vi "Add_Shortcut.vi"(8 "error in (no error)":errorcluster, 9 "shortcutAddresses":T1[](array[typedef]), 10 "shortcut":refnum<class "IB_Shortcut.lvclass">, 11 "IB_Source in":refnum<class "IB_Source.lvclass">) -> (0 "error out":errorcluster, 1 "name change?":bool, 2 "shortcut":refnum<class "IB_Shortcut.lvclass">, 3 "IB_Source out":refnum<class "IB_Source.lvclass">)   [LabVIEW 2020, in "IB_Source.lvclass"]
uses:
  <vilib>/AppBuilder/IB_Classes/Source/IB_Source.lvclass
  <vilib>/AppBuilder/IB_Classes/Source/IB_Source.lvclass/IB_Source.ctl
  <vilib>/AppBuilder/IB_Classes/Shortcut/IB_Shortcut.lvclass
  <resource>/Framework/Providers/Builds/Installer/CDK_sTypeDef_ShortcutAddress.ctl
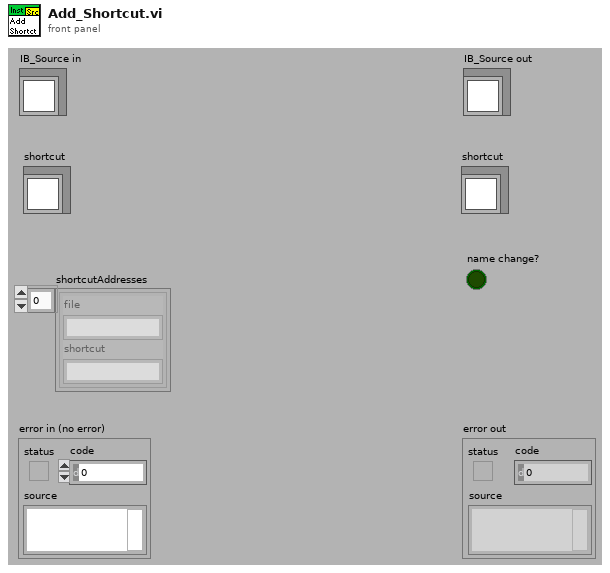
[diagram p1: front panel]
types:
  T1 = typedef "CDK_sTypeDef_ShortcutAddress.ctl" = cluster{"file":string, "shortcut":string}
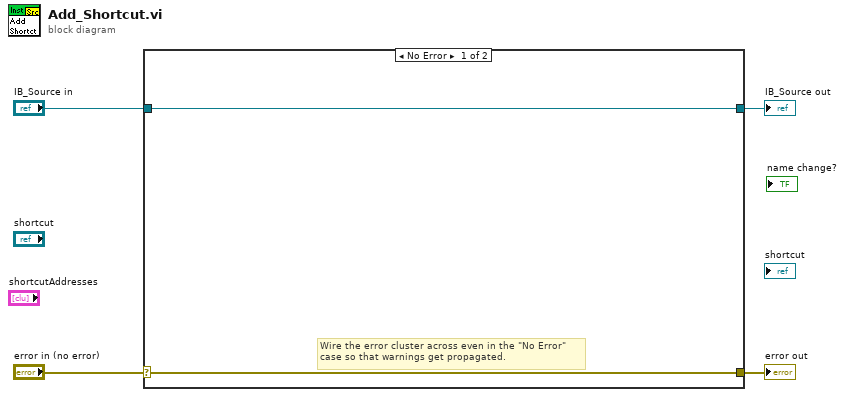
[diagram p0: block diagram]
diagram:
  n1 = case shown="No Error" "error in (no error)" {
    selector: "error in (no error)" -> [w5 w8]
    tunnel: [w5 w8] -> w3
    tunnel: [w6 w7] -> w1
    tunnel: "IB_Source in" -> [w6 w7]
    frame No Error {
      # "Wire the error cluster across even in the \"No Error\"\ncase so that warnings get propagated."
    }
    frame Error {
    }
  }
  "error out" <- w3
  "IB_Source out" <- w1
